vi "Program02.vi"() -> ()   [LabVIEW 2015]
uses:
  <vilib>/measure/NI_MABase.lvlib
panel:
  out "m2":dynamicdata(graph)
  out "m1":dynamicdata(graph)
  out "detected m2":dynamicdata(graph)
  out "detected m1":dynamicdata(graph)
  in  "sampling info 4":cluster{"Fs":dbl, "#s":dbl}={"Fs"=1000.0, "#s"=1000.0} {"Fs" format="%.2p"}
  in  "seed 2":i32=-1
  in  "sampling info 3":cluster{"Fs":dbl, "#s":dbl}={"Fs"=1000.0, "#s"=1000.0} {"Fs" format="%.2p"}
  in  "seed":i32=-1
  in  "sampling info 2":cluster{"Fs":dbl, "#s":dbl}={"Fs"=1000.0, "#s"=1000.0} {"Fs" format="%.2p"}
  in  "signal type 2":T1(ring)
  in  "phase 2":dbl format="%.2p"
  in  "amplitude 2":dbl=1.0 format="%0.2p"
  in  "frequency 2":dbl=10.0 format="%0.2p"
  in  "sampling info":cluster{"Fs":dbl, "#s":dbl}={"Fs"=1000.0, "#s"=1000.0} {"Fs" format="%.2p"}
  in  "signal type":T1(ring)
  in  "phase":dbl format="%.2p"
  in  "amplitude":dbl=1.0 format="%0.2p"
  in  "frequency":dbl=10.0 format="%0.2p"
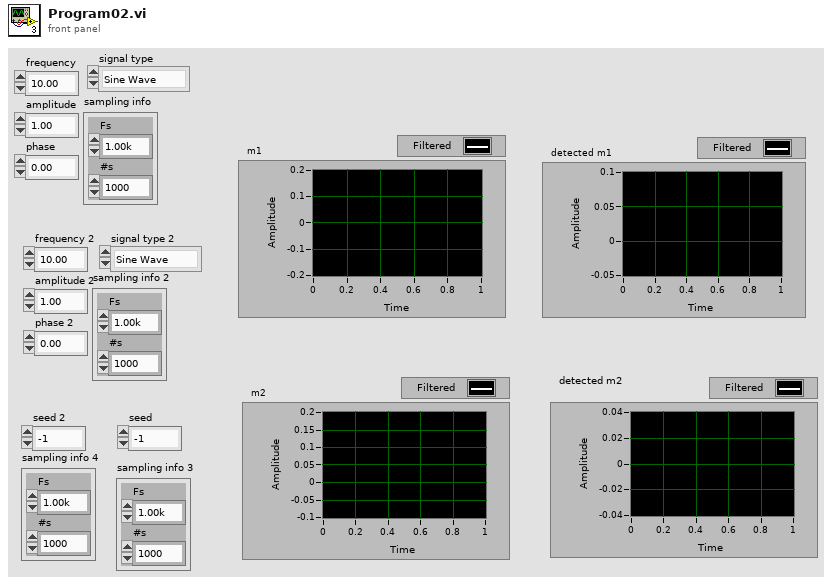
[diagram p1: front panel]
types:
  T1 = enum16{"Sine Wave", "Triangle Wave", "Square Wave", "Sawtooth Wave"}
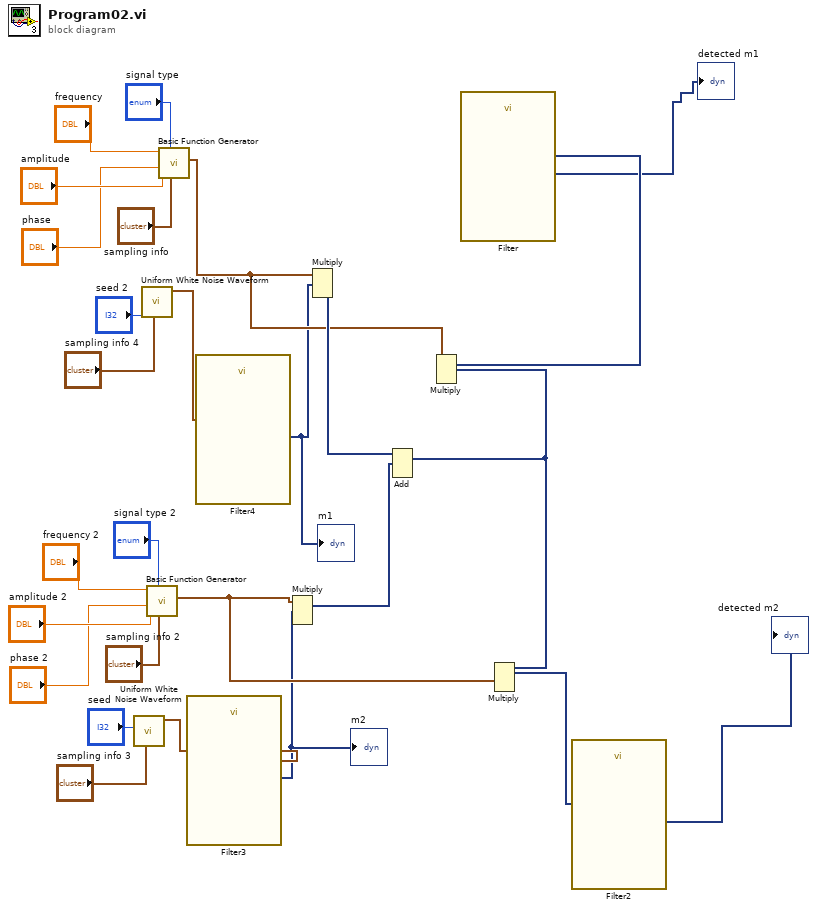
[diagram p0: block diagram]
diagram:
  n1 = call <vilib>:"Uniform White Noise Waveform.vi"("sampling info"="sampling info 3", "seed"="seed") -> ("signal out"=w6:waveform(dbl))  [unwired: 8 in, 1 out]
  n2 = call <vilib>:"Uniform White Noise Waveform.vi"("sampling info"="sampling info 4", "seed"="seed 2") -> ("signal out"=w5:waveform(dbl))  [unwired: 8 in, 1 out]
  n3 = call <vilib>:"Basic Function Generator.vi"("sampling info"="sampling info 2", "signal type"="signal type 2", "phase"="phase 2", "amplitude"="amplitude 2", "frequency"="frequency 2") -> ("signal out"=w10:waveform(dbl))  [unwired: 4 in, 2 out]
  n4 = call <vilib>:"Basic Function Generator.vi"("sampling info"="sampling info", "signal type"="signal type", "phase"="phase", "amplitude"="amplitude", "frequency"="frequency") -> ("signal out"=w9:waveform(dbl))  [unwired: 4 in, 2 out]
  n5 = call "Filter3"("Signal"=w6) -> ("Filtered Signal"=w3:dynamicdata)  [unwired: 9 in, 1 out]
  "m2" <- w3
  n6 = call "Filter4"("Signal"=w5) -> ("Filtered Signal"=w4:dynamicdata)  [unwired: 9 in, 1 out]
  "m1" <- w4
  n7 = Multiply(1:w3, 2:w10) -> (0:w12:dynamicdata)  [unwired: 1 in, 1 out]
  n8 = Multiply(1:w4, 2:w9) -> (0:w13:dynamicdata)  [unwired: 1 in, 1 out]
  n9 = Add(1:w12, 2:w13) -> (0:w11:dynamicdata)  [unwired: 1 in, 1 out]
  n10 = Multiply(1:w11, 2:w9) -> (0:w8:dynamicdata)  [unwired: 1 in, 1 out]
  n11 = call "Filter"("Signal"=w8) -> ("Filtered Signal"=→"detected m1":dynamicdata)  [unwired: 9 in, 1 out]
  n12 = Multiply(1:w10, 2:w11) -> (0:w2:dynamicdata)  [unwired: 1 in, 1 out]
  n13 = call "Filter2"("Signal"=w2) -> ("Filtered Signal"=→"detected m2":dynamicdata)  [unwired: 9 in, 1 out]
